vi "TCP Command Parse New.vi"(1 "Command Msg":string, 3 "SetChNums":T1) -> (14 "ADChannelStructArray":T4, 15 "DAChannelStructArray":T2)   [LabVIEW 2011]
doc: "Reads an incoming package of data from a remote host via TCP/IP. This VI parses the package and extracts the data name and type as described in the meta data.\n\nFor the package to be parsed correctly, the meta data must be consistent in both the sender and the receiver. The data is packaged based on the existing meta data on the sender. Inconsistent meta data will result in inconsistent data parsing.\nUse the \"Read Meta\" and \"Write Meta\" VIs to ensure that both client and server have the same meta data.\n\nThe data is returned as a string. It is the responsibility of the user to cast it to the appropriate type before usage."
uses:
  ADChannelStructArray.ctl
  ADChannelStruct.ctl
  DAChannelStructArray.ctl
  DAChannelStruct.ctl
  CommandFrameHead.ctl
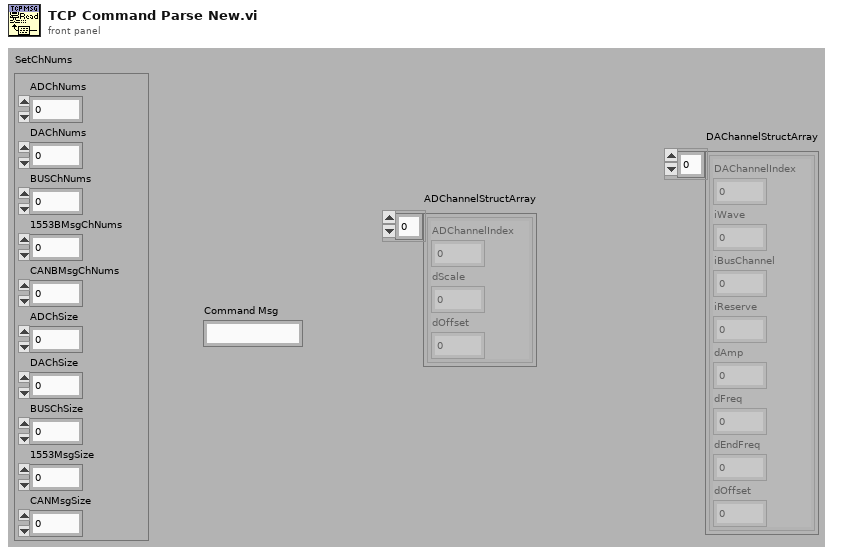
[diagram p1: front panel]
types:
  T1 = typedef "CommandFrameHead.ctl" = cluster{"ADChNums":i32, "DAChNums ":i32, "BUSChNums":i32, "1553BMsgChNums":i32, "CANBMsgChNums ":i32, "ADChSize":i32, "DAChSize":i32, "BUSChSize":i32, "1553MsgSize":i32, "CANMsgSize":i32}
  T2 = typedef "DAChannelStructArray.ctl" = T3[]
  T3 = typedef "DAChannelStruct.ctl" = cluster{"DAChannelIndex":i32, "iWave":i32, "iBusChannel":i32, "iReserve":i32, "dAmp":dbl, "dFreq":dbl, "dEndFreq":dbl, "dOffset":dbl}
  T4 = typedef "ADChannelStructArray.ctl" = T5[]
  T5 = typedef "ADChannelStruct.ctl" = cluster{"ADChannelIndex":i32, "dScale":dbl, "dOffset":dbl}
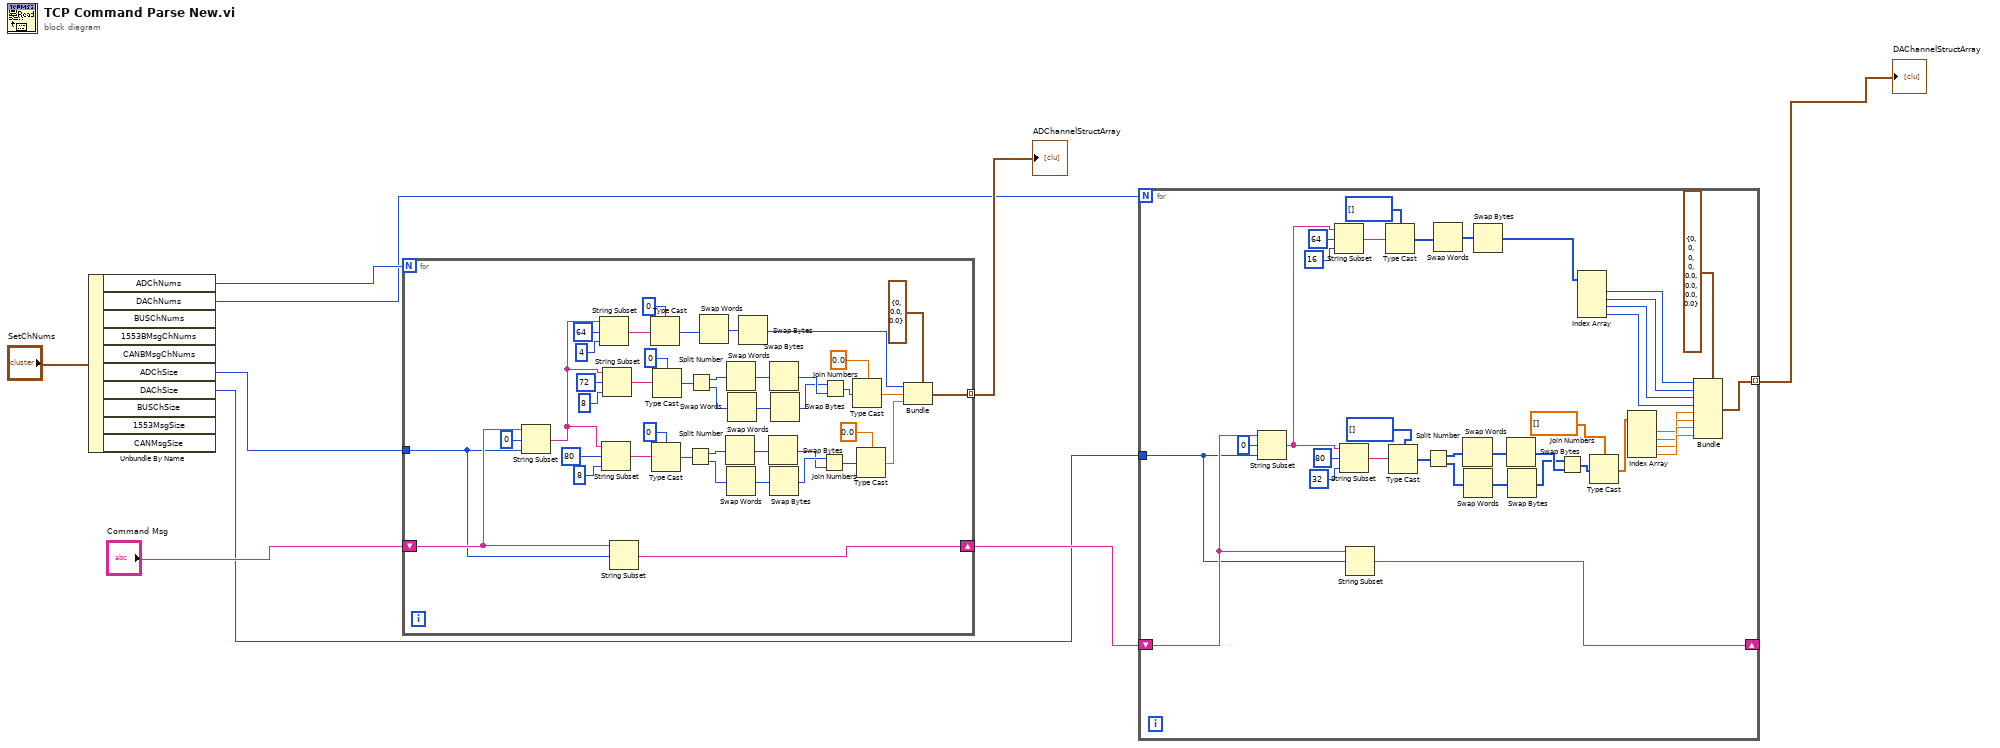
[diagram p0: block diagram]
diagram:
  n1 = Unbundle By Name("SetChNums") -> ("ADChNums"=w8:i32, "DAChNums"=w5:i32, "ADChSize"=w2:i32, "DAChSize"=w1:i32)  [unwired: 6 out]
  n2 = for {
    N: w8 -> [_]
    shift-right: [w48] -> w6
    shift-left: "Command Msg" -> [w49]
    tunnel: w2 -> [w21]
    tunnel: [w12] -> w7 mode=indexing
    n3 = String Subset(string=w49, offset (0)=0, length (rest)=w21) -> (substring=w23:string)
    n4 = String Subset(string=w23, offset (0)=64, length (rest)=4 ("length (rest)")) -> (substring=w43:string)
    n5 = String Subset(string=w23, offset (0)=80, length (rest)=8 ("length (rest)")) -> (substring=w25:string)
    n6 = String Subset(string=w23, offset (0)=72, length (rest)=8 ("length (rest)")) -> (substring=w40:string)
    n7 = String Subset(string=w49, offset (0)=w21) -> (substring=w48:string)  [unwired: 1 in]
    n8 = Type Cast(type=0 ("bytes to read"), x=w43) -> (*(type *) &x=w42:i32)
    n9 = Type Cast(type=i64 0 ("bytes to read"), x=w25) -> (*(type *) &x=w32:i64)
    n10 = Type Cast(type=i64 0 ("bytes to read"), x=w40) -> (*(type *) &x=w33:i64)
    n11 = Split Number(x=w32) -> (hi(x)=w27:u32, lo(x)=w29:u32)
    n12 = Split Number(x=w33) -> (hi(x)=w38:u32, lo(x)=w36:u32)
    n13 = Swap Words(1:w42) -> (0:w50:i32)
    n14 = Swap Words(1:w27) -> (0:w26:u32)
    n15 = Swap Words(1:w38) -> (0:w39:u32)
    n16 = Swap Words(1:w29) -> (0:w28:u32)
    n17 = Swap Words(1:w36) -> (0:w37:u32)
    n18 = Swap Bytes(anything=w50) -> (byte swapped=w19:i32)
    n19 = Swap Bytes(anything=w26) -> (byte swapped=w30:u32)
    n20 = Swap Bytes(anything=w39) -> (byte swapped=w35:u32)
    n21 = Swap Bytes(anything=w28) -> (byte swapped=w31:u32)
    n22 = Swap Bytes(anything=w37) -> (byte swapped=w34:u32)
    n23 = Join Numbers(hi=w31, lo=w30) -> ((hi.lo)=w14:u64)
    n24 = Join Numbers(hi=w34, lo=w35) -> ((hi.lo)=w18:u64)
    n25 = Type Cast(type=0.0 ("bytes to read"), x=w18) -> (*(type *) &x=w17:dbl)
    n26 = Type Cast(type=0.0 ("bytes to read"), x=w14) -> (*(type *) &x=w13:dbl)
    n27 = Bundle(cluster=T5 {"ADChannelIndex"=0, "dScale"=0.0, "dOffset"=0.0} ("ADChannelStruct"), "ADChannelIndex"=w19, "dScale"=w17, "dOffset"=w13) -> (w12:T5)
  }
  "ADChannelStructArray" <- w7
  n28 = for {
    N: w5 -> [_]
    shift-right: [w84] -> _
    shift-left: w6 -> [w85]
    tunnel: w1 -> [w70]
    tunnel: [w63] -> w4 mode=indexing
    n29 = String Subset(string=w85, offset (0)=0, length (rest)=w70) -> (substring=w58:string)
    n30 = String Subset(string=w58, offset (0)=64, length (rest)=16 ("length (rest)")) -> (substring=w80:string)
    n31 = String Subset(string=w58, offset (0)=80, length (rest)=32 ("length (rest)")) -> (substring=w78:string)
    n32 = String Subset(string=w85, offset (0)=w70) -> (substring=w84:string)  [unwired: 1 in]
    n33 = Type Cast(type=i32[] [], x=w80) -> (*(type *) &x=w79:i32[])
    n34 = Type Cast(type=i64[] [], x=w78) -> (*(type *) &x=w71:i64[])
    n35 = Split Number(x=w71) -> (hi(x)=w76:u32[], lo(x)=w74:u32[])
    n36 = Swap Words(1:w79) -> (0:w86:i32[])
    n37 = Swap Words(1:w76) -> (0:w77:u32[])
    n38 = Swap Words(1:w74) -> (0:w75:u32[])
    n39 = Swap Bytes(anything=w86) -> (byte swapped=w56:i32[])
    n40 = Swap Bytes(anything=w77) -> (byte swapped=w73:u32[])
    n41 = Swap Bytes(anything=w75) -> (byte swapped=w72:u32[])
    n42 = Join Numbers(hi=w72, lo=w73) -> ((hi.lo)=w68:u64[])
    n43 = Index Array(array=w56) -> (element #1=w55:i32, element #2=w54:i32, element #3=w53:i32, element #4=w52:i32)  [unwired: 4 in]
    n44 = Type Cast(type=dbl[] [], x=w68) -> (*(type *) &x=w64:dbl[])
    n45 = Index Array(array=w64) -> (element #1=w59:dbl, element #2=w60:dbl, element #3=w61:dbl, element #4=w62:dbl)  [unwired: 4 in]
    n46 = Bundle(cluster=T3 {"DAChannelIndex"=0, "iWave"=0, "iBusChannel"=0, "iReserve"=0, "dAmp"=0.0, "dFreq"=0.0, "dEndFreq"=0.0, "dOffset"=0.0} ("DAChannelStruct"), "DAChannelIndex"=w55, "iWave"=w54, "iBusChannel"=w53, "iReserve"=w52, "dAmp"=w59, "dFreq"=w60, "dEndFreq"=w61, "dOffset"=w62) -> (w63:T3)
  }
  "DAChannelStructArray" <- w4
